vi "Find XML Descriptor.vi"(8 "error in":errorcluster, 11 "Project Path":path) -> (0 "error out":errorcluster, 2 "Found ?":bool, 3 "XML Path":path, 5 "Custom Device Name":string, 7 "Common Doc Dir":string)   [LabVIEW 2018, in ".LVLIBP CD XML Updater.lvlib" / "Project XML Editor.lvclass"]
uses:
  Project XML Editor.lvclass
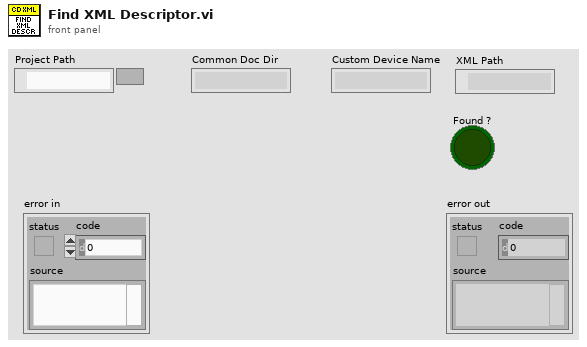
[diagram p1: front panel]
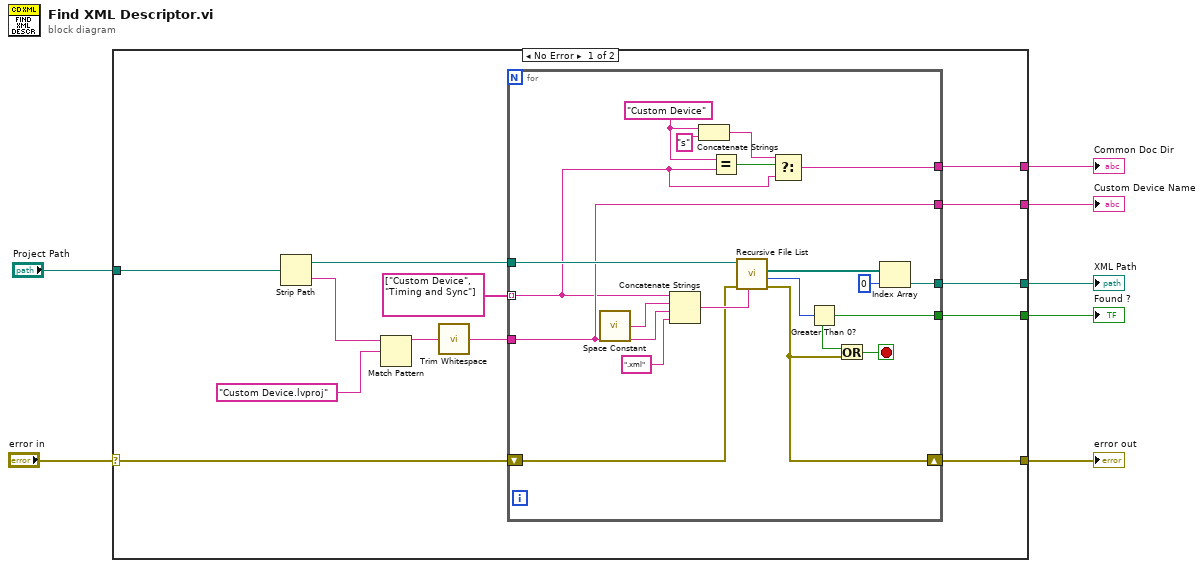
[diagram p0: block diagram]
diagram:
  n1 = case shown="No Error" "error in" {
    selector: "error in" -> [w12 w40]
    tunnel: "Project Path" -> [w14 _]
    tunnel: [w13 _] -> w6
    tunnel: [w11 w40] -> w4
    tunnel: [w10 _] -> w3
    tunnel: [w9 _] -> w2
    tunnel: [w8 _] -> w1
    frame No Error {
      n2 = Strip Path(path=w14) -> (stripped path=w17:path, name=w15:string)
      n3 = Match Pattern(string=w15, regular expression="Custom Device.lvproj") -> (before substring=w19:string)  [unwired: 1 in, 3 out]
      n4 = call <vilib>:"Trim Whitespace.vi"("string"=w19) -> ("trimmed string"=w20:string)  [unwired: 1 in]
      n5 = for {
        tunnel: w17 -> [w37]
        tunnel: string[] ["Custom Device", "Timing and Sync"] -> [w22] mode=indexing
        tunnel: w20 -> [w27]
        tunnel: [w31] -> w13
        tunnel: [w30] -> w10
        shift-right: [w28] -> w11
        shift-left: w12 -> [w29]
        tunnel: [w27] -> w9
        tunnel: [w21] -> w8
        stop <- w34 stop-if-true
        w25 = "Custom Device" ("y")
        n6 = call <vilib>:"Space Constant.vi"() -> ("String"=w38:string)
        n7 = Concatenate Strings(w22, w38, w27, ".xml" ("string")) -> (w36:string)
        n8 = Concatenate Strings(w25, "s" ("string")) -> (w23:string)
        n9 = Equal?(x=w25, y=w22) -> (x = y?=w26:bool)
        n10 = call <vilib>:"Recursive File List.vi"("pattern"=w36, "error in (no error)"=w29, "Folder Path"=w37) -> ("error out"=w28:errorcluster, "Number of Files"=w35:i32, "All Files in Dir"=w33:path[])  [unwired: 4 in, 2 out]
        n11 = Select(t=w23, s=w26, f=w22) -> (s? t:f=w21:string)
        n12 = Greater Than 0?(x=w35) -> (x > 0?=w30:bool)
        n13 = Or(x=w30, y=w28) -> (x .or. y?=w34:bool)
        n14 = Index Array(array=w33, index=0) -> (element=w31:path)
      }
    }
    frame Error {
    }
  }
  "XML Path" <- w6
  "error out" <- w4
  "Found ?" <- w3
  "Custom Device Name" <- w2
  "Common Doc Dir" <- w1
